vi "PointToRotateRectangel.vi"(8 "error in":errorcluster, 9 "rotate":dbl, 10 "Size":cluster{"Width":sgl, "Height":sgl} {"Height" format="%.2f"; "Width" format="%.2f"}, 11 "Center Point":T1 {"Y" format="%.2f"; "X" format="%.2f"}) -> (0 "error out":errorcluster, 3 "Output Points":T1[](array[typedef]) {"Y" format="%.2f"; "X" format="%.2f"})   [LabVIEW 2015]
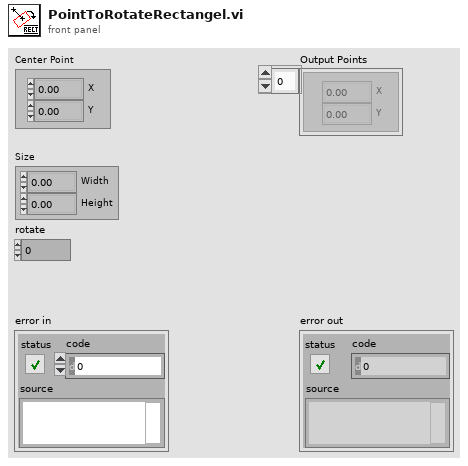
[diagram p1: front panel]
types:
  T1 = typedef "IMAQ Point" = cluster{"X":sgl, "Y":sgl}
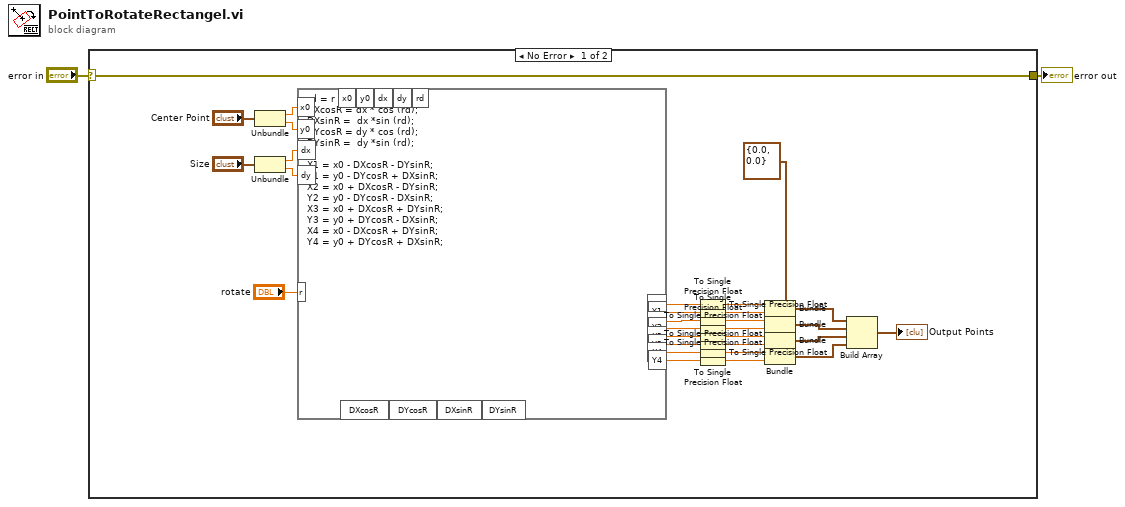
[diagram p0: block diagram]
diagram:
  n1 = case shown="No Error" "error in" {
    selector: "error in" -> [w24 w33]
    tunnel: [w24 w33] -> w1
    frame No Error {
      w23 = T1 {"X"=0.0, "Y"=0.0} ("Center Point 2")
      n2 = Unbundle("Center Point") -> ("X"=w30:sgl, "Y"=w31:sgl)
      n3 = Unbundle("Size") -> ("Width"=w28:sgl, "Height"=w27:sgl)
      n4 = formula code="rd = r * pi / 180.0;\nDXcosR = dx * cos (rd);\nDXsinR =  dx *sin (rd);\nDYcosR = dy * cos (rd);\nDYsinR =  dy *sin (rd);\n\nX1 = x0 - DXcosR - DYsinR;\nY1 = y0 - DYcosR + DXsinR;\nX2 = x0 + DXcosR - DYsinR;\nY2 = y0 - DYcosR - DXsinR;\nX3 = x0 + DXcosR + DYsinR;\nY3 = y0 + DYcosR - DXsinR;\nX4 = x0 - DXcosR + DYsinR;\nY4 = y0 + DYcosR + DXsinR;"("r"="rotate", "x0"=w30, "y0"=w31, "dx"=w28, "dy"=w27) -> ("X1"=w22:dbl, "Y1"=w13:dbl, "X2"=w12:dbl, "Y2"=w11:dbl, "X3"=w10:dbl, "Y3"=w9:dbl, "X4"=w8:dbl, "Y4"=w7:dbl)  [unwired: 9 out]
      n5 = To Single Precision Float(number=w22) -> (single precision float=w21:sgl)
      n6 = To Single Precision Float(number=w13) -> (single precision float=w15:sgl)
      n7 = To Single Precision Float(number=w12) -> (single precision float=w14:sgl)
      n8 = To Single Precision Float(number=w11) -> (single precision float=w20:sgl)
      n9 = To Single Precision Float(number=w10) -> (single precision float=w19:sgl)
      n10 = To Single Precision Float(number=w9) -> (single precision float=w18:sgl)
      n11 = To Single Precision Float(number=w8) -> (single precision float=w17:sgl)
      n12 = To Single Precision Float(number=w7) -> (single precision float=w16:sgl)
      n13 = Bundle(cluster=w23, "X"=w21, "Y"=w15) -> (w6:T1)
      n14 = Bundle(cluster=w23, "X"=w14, "Y"=w20) -> (w5:T1)
      n15 = Bundle(cluster=w23, "X"=w19, "Y"=w18) -> (w4:T1)
      n16 = Bundle(cluster=w23, "X"=w17, "Y"=w16) -> (w3:T1)
      n17 = Build Array(w6, w5, w4, w3) -> (→"Output Points":T1[])
    }
    frame Error {
    }
  }
  "error out" <- w1
